vi "arduinoInitSerial.vi"(1 "Serial Settings:Baud Rate":u32=2400, 2 "VISA resource name":refnum<visa-resource-name>="COM3") -> (0 "serial status":u32(colorbox)=6618880)   [LabVIEW 2012]
uses:
  <vilib>/Instr/_visa.llb/VISA Set IO Buffer Mask.ctl
  <vilib>/Instr/_visa.llb/VISA Configure Serial Port (Instr).vi
  GlobalArduino.vi
panel:
  out "error out":errorcluster
  in  "size (4096)":u32=4096
  in  "Mask":T1=16 items=["I/O Receive Buffer"=16, "I/O Transmit Buffer"=32, "I/O Receive and Transmit Buffer"=48]
  in  "Enable Termination\nChar (T)":bool=TRUE
  in  "termination char\n(0xD)":u8=13 format="%.0x"
  in  "timeout (10sec)":u32=10000
  in  "parity (0:none)":enum16{"None", "Odd", "Even", "Mark", "Space"}(ring)
  in  "Serial Settings:End Mode for Writes":u16(ring)=2 items=["None", "Last Bit", "TermChar", "Break"]
  in  "Serial Settings:Flow Control":u16(ring) items=["None", "XON/XOFF", "RTS/CTS", "XON/XOFF & RTS/CTS", "DTR/DSR", "XON/XOFF & DTR/DSR"]
  in  "Serial Settings:Stop Bits":u16(ring)=10 items=["1.0"=10, "1.5"=15, "2.0"=20]
  in  "Serial Settings:Data Bits":u16=8
  in  "Serial Settings:Modem Line Settings:Line DTR State":i16(ring) items=["Unknown"=-1, "Unasserted"=0, "Asserted"=1]
  in  "Serial Settings:Modem Line Settings:Line RTS State":i16(ring) items=["Unknown"=-1, "Unasserted"=0, "Asserted"=1]
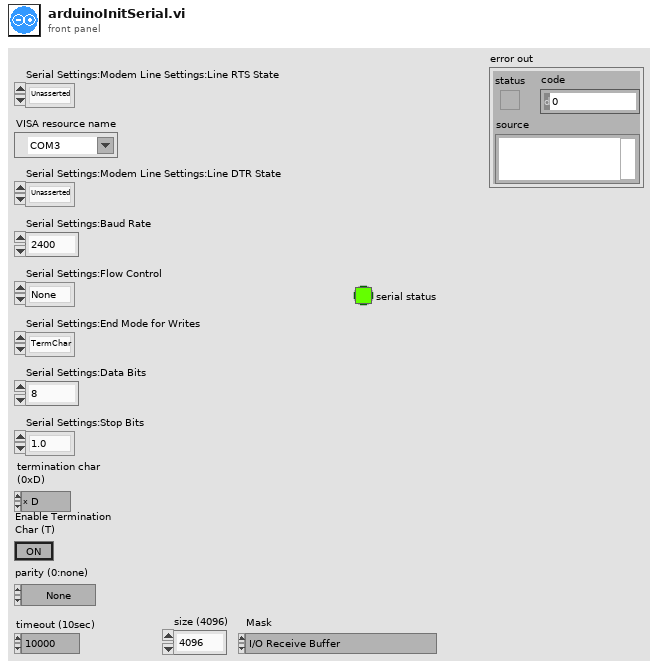
[diagram p1: front panel]
types:
  T1 = typedef "VISA Set IO Buffer Mask.ctl" = u16
  T2 = typedef "Semaphore RefNum" = refnum<k1>
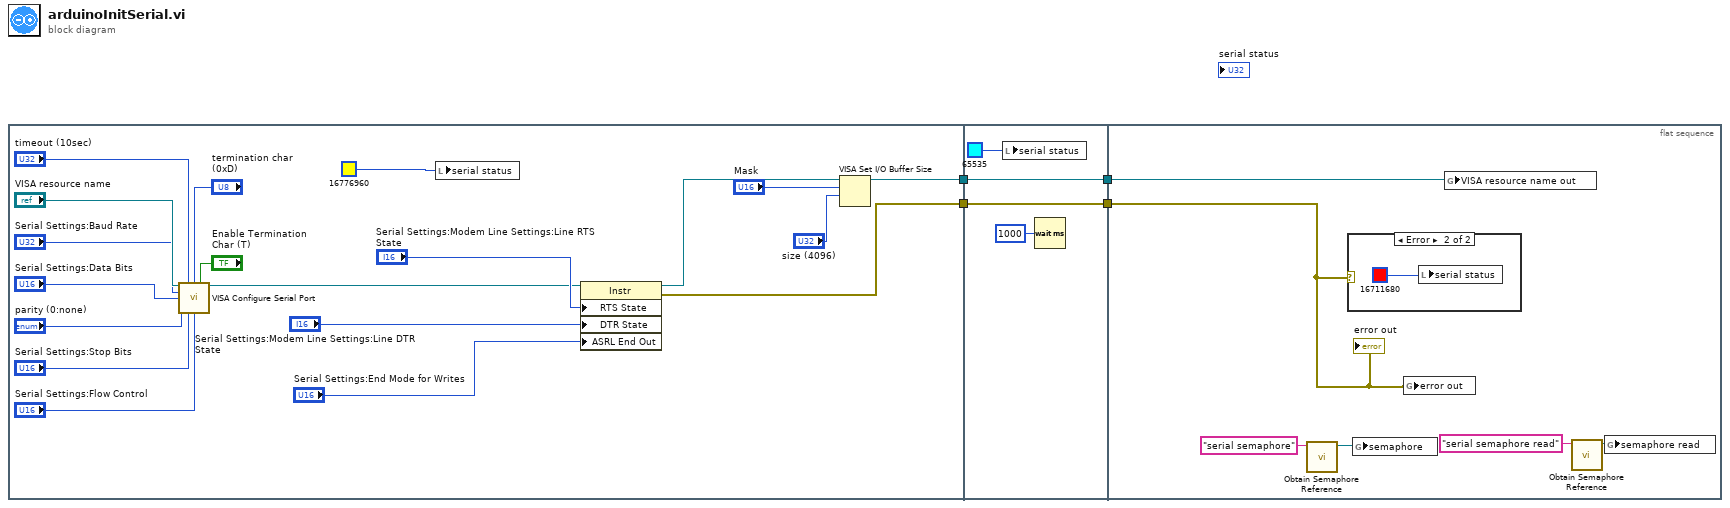
[diagram p0: block diagram]
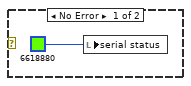
[diagram p2: hidden frame]
diagram:
  n1 = flat-sequence {
    tunnel: [w6] -> w2
    tunnel: [w5] -> w1
    tunnel: [w24] -> w4
    tunnel: [w25] -> w3
    tunnel: w2 -> [w25]
    tunnel: w1 -> [w24]
    tunnel: w4 -> [w30]
    tunnel: w3 -> [w31]
    frame #0 {
      n2 = call-poly "VISA Configure Serial Port"("VISA resource name"="VISA resource name", "timeout (10sec)"="timeout (10sec)", "termination char\n(0xA = '\\n' = LF)"="termination char\n(0xD)", "Enable Termination\nChar (T)"="Enable Termination\nChar (T)", "baud rate (9600)"="Serial Settings:Baud Rate", "data bits (8)"="Serial Settings:Data Bits", "parity (0:none)"="parity (0:none)", "stop bits (10: 1 bit)"="Serial Settings:Stop Bits", "flow control (0:none)"="Serial Settings:Flow Control") -> ("VISA resource name out"=w11:refnum<visa-resource-name>)  [unwired: 5 in, 1 out]
      n3 = local write "serial status"(u32 16776960 ("Unit_Condition")) -> ()
      n4 = property class="Instr"(reference=w11, "RTS State"="Serial Settings:Modem Line Settings:Line RTS State", "DTR State"="Serial Settings:Modem Line Settings:Line DTR State", "ASRL End Out"="Serial Settings:End Mode for Writes") -> (reference out=w9:refnum<visa-resource-name>, error out=w5:errorcluster)  [unwired: 1 in]
      n5 = VISA Set I/O Buffer Size(VISA resource name=w9, mask (16)="Mask", size (4096)="size (4096)") -> (VISA resource name out=w6:refnum<visa-resource-name>)  [unwired: 1 in, 1 out]
    }
    frame #1 {
      n6 = local write "serial status"(u32 65535 ("Unit_Condition")) -> ()
      n7 = Wait (ms)(milliseconds to wait=u32 1000) -> ()  [unwired: 1 out]
    }
    frame #2 {
      n8 = call <vilib>:"Obtain Semaphore Reference.vi"("name (unnamed)"="serial semaphore") -> ("semaphore"=w32:T2)  [unwired: 4 in, 2 out]
      n9 = case shown="Error" w30 {
        frame No Error {
          n10 = local write "serial status"(u32 6618880 ("Unit_Condition")) -> ()
        }
        frame Error {
          n11 = local write "serial status"(u32 16711680 ("Unit_Condition")) -> ()
        }
      }
      n12 = global write "GlobalArduino.vi" "semaphore"(w32) -> ()
      n13 = global write "GlobalArduino.vi" "error out"(w30) -> ()
      n14 = global write "GlobalArduino.vi" "VISA resource name out"(w31) -> ()
      n15 = call <vilib>:"Obtain Semaphore Reference.vi"("name (unnamed)"="serial semaphore read") -> ("semaphore"=w28:T2)  [unwired: 4 in, 2 out]
      n16 = global write "GlobalArduino.vi" "semaphore read"(w28) -> ()
      "error out" <- w30
    }
  }
